vi "Jog data test.vi"() -> ()   [LabVIEW 2016]
panel:
  in  "Jog Cluster":T1={"Jog XY Cluster"={"object goes up"=FALSE, "object goes down"=FALSE, "object goes right"=FALSE, "object goes left"=FALSE, "SW2"=FALSE, "SW1"=FALSE, "YY (mm)"=0.1, "YN (mm) "=0.01, "NY (mm) "=0.005, "NN (mm) "=0.001}, "Jog Z Cluster "={"Z go down 0.1 mm"=FALSE, "Z go up 0.1 mm"=FALSE, "Z go down 0.05 mm"=FALSE, "Z go up 0.05 mm"=FALSE, "Z go down 0.01 mm"=FALSE, "Z go up 0.01 mm"=FALSE, "Z go down"=FALSE, "Z go up"=FALSE, "step (mm)"=0.001}}
  out "array OUT":dbl[](array[numeric])
  in  "array IN":dbl[](array[numeric])
  in  "stop":bool
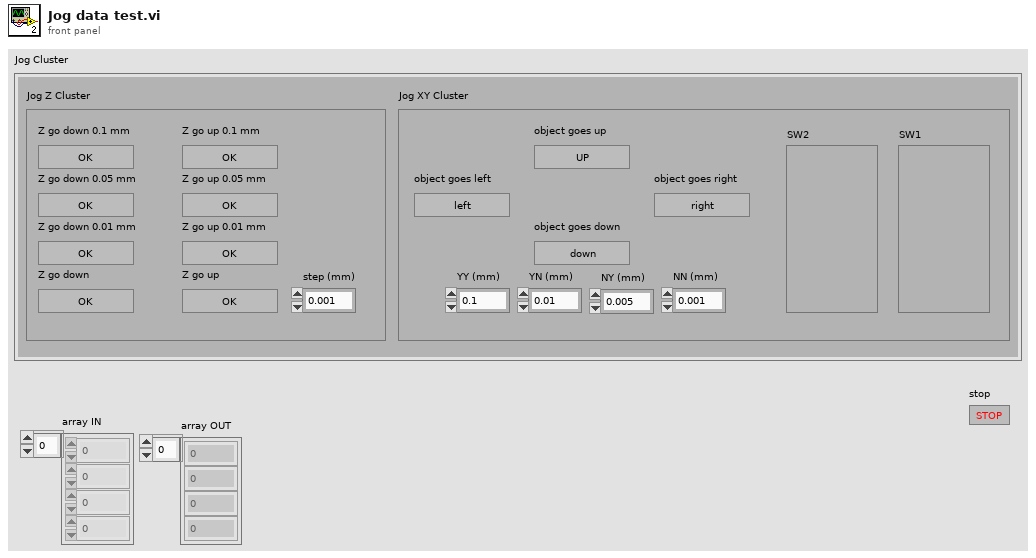
[diagram p1: front panel]
types:
  T1 = cluster{"Jog XY Cluster":cluster{"object goes up":bool, "object goes down":bool, "object goes right":bool, "object goes left":bool, "SW2":bool, "SW1":bool, "YY (mm)":dbl, "YN (mm) ":dbl, "NY (mm) ":dbl, "NN (mm) ":dbl}, "Jog Z Cluster ":cluster{"Z go down 0.1 mm":bool, "Z go up 0.1 mm":bool, "Z go down 0.05 mm":bool, "Z go up 0.05 mm":bool, "Z go down 0.01 mm":bool, "Z go up 0.01 mm":bool, "Z go down":bool, "Z go up":bool, "step (mm)":dbl}}
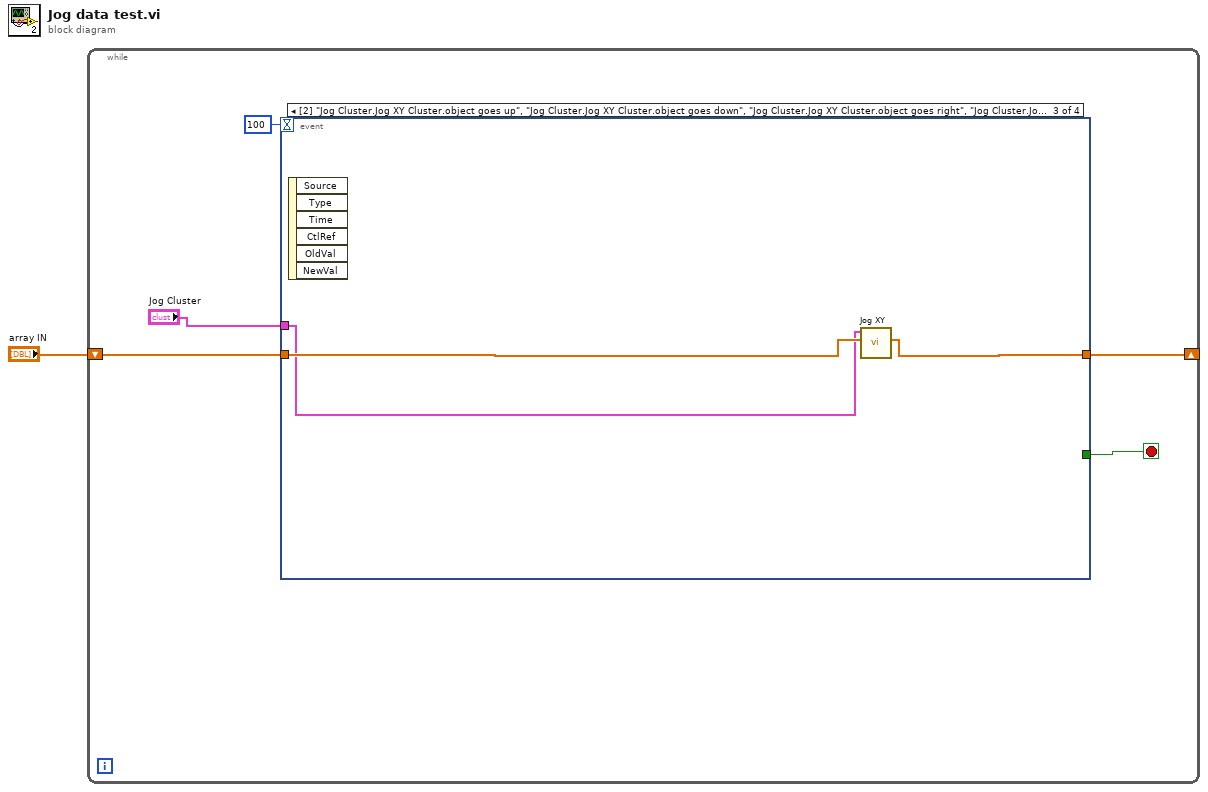
[diagram p0: block diagram]
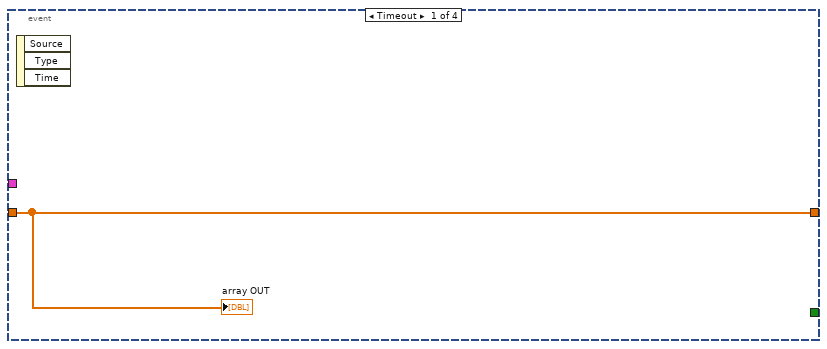
[diagram p2: hidden frame]
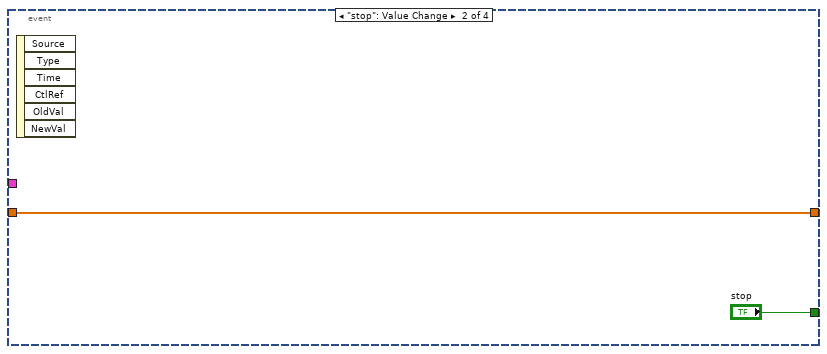
[diagram p3: hidden frame]
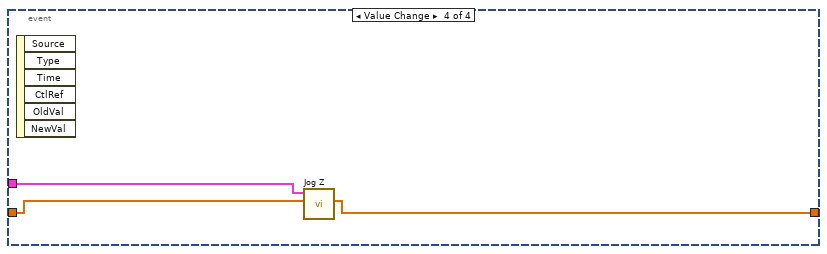
[diagram p4: hidden frame]
diagram:
  n1 = while {
    shift-right: [w3] -> _
    shift-left: "array IN" -> [w4]
    stop <- w5 stop-if-true
    n2 = event shown="[2] \"Jog Cluster.Jog XY Cluster.object goes up\", \"Jog Cluster.Jog XY Cluster.object goes down\", \"Jog Cluster.Jog XY Cluster.object goes right\", \"Jog Cluster.Jog XY Cluster.object goes left\": Value Change" {
      selector: _ -> [_ _ _ _]
      dyn-events: _ -> [_ _ _ _]
      timeout: 100 -> [_ _ _ _]
      tunnel: [_ "stop" _ _] -> w5
      tunnel: w4 -> [w7 w8 w12 w15]
      tunnel: [w7 w8 w11 w14] -> w3
      tunnel: "Jog Cluster" -> [_ _ w10 w13]
      event Timeout {
        n3 = event-data() -> ()  [unwired: 1 in, 3 out]
        "array OUT" <- w7
      }
      event "stop": Value Change {
        n4 = event-data() -> ()  [unwired: 1 in, 6 out]
      }
      event "Jog Cluster.Jog XY Cluster.object goes up", "Jog Cluster.Jog XY Cluster.object goes down", "Jog Cluster.Jog XY Cluster.object goes right", "Jog Cluster.Jog XY Cluster.object goes left": Value Change {
        n5 = event-data() -> ()  [unwired: 1 in, 6 out]
        n6 = call "Jog XY.vi"("array IN"=w12, "Jog Cluster"=w10) -> ("array OUT"=w11:dbl[])  [unwired: 8 in, 1 out]
      }
      event "Jog Cluster.Jog Z Cluster.Z go down 0.1 mm", "Jog Cluster.Jog Z Cluster.Z go up 0.1 mm", "Jog Cluster.Jog Z Cluster.Z go down 0.05 mm", "Jog Cluster.Jog Z Cluster.Z go up 0.05 mm", "Jog Cluster.Jog Z Cluster.Z go down 0.01 mm", "Jog Cluster.Jog Z Cluster.Z go up 0.01 mm", "Jog Cluster.Jog Z Cluster.Z go down", "Jog Cluster.Jog Z Cluster.Z go up": Value Change {
        n7 = event-data() -> ()  [unwired: 1 in, 6 out]
        n8 = call "Jog Z.vi"("array IN"=w15, "Jog Cluster"=w13) -> ("array OUT"=w14:dbl[])  [unwired: 8 in, 1 out]
      }
    }
  }
